vi "Create TCP Slave.vi"(8 "error in":errorcluster, 10 "port (502)":u16=502, 11 "address":string) -> (0 "error out":errorcluster, 3 "TCP slave instance":refnum<class "Modbus Slave.lvclass">)   [LabVIEW 2013, in "Modbus Library - Advance.lvlib" / "API Main.lvlib"]
doc: "Creates a standard TCP slave with an IP ADU. If the data model input is unwired, a standard data model will be initialized and used. If the input is wired, the code will check to make sure that it is not the default value for the class (it should be initialized). If the default value of the class is wired, the standard model will be initialized and used."
uses:
  API Main.lvlib
  Slave/Modbus Slave.lvclass
  Transmission Data Unit/IP/IP Data Unit.lvclass
  Network Protocol/Network Slave/TCP/TCP Slave.lvclass
  Transmission Data Unit/Transmission Data Unit.lvclass/Transmission Data Unit.ctl
  Super Data Model/Super Data Model.lvclass
  Network Protocol/Network Slave/TCP/TCP Slave.lvclass/TCP Slave.ctl
  Slave/Modbus Slave.lvclass/Modbus Slave.ctl
  Modbus API.lvclass/Modbus API.ctl
  Network Protocol/Network Slave/TCP/Write Port.vi
  Network Protocol/Network Slave/TCP/Write listening net address.vi
  <vilib>/Utility/error.llb/Clear Errors.vi
  Super Data Model/ShutDown.vi
  Modbus API.lvclass
  Transmission Data Unit/Transmission Data Unit.lvclass
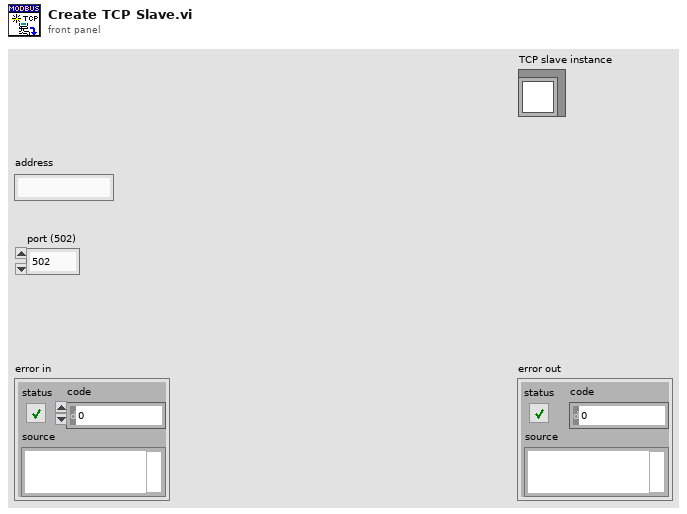
[diagram p1: front panel]
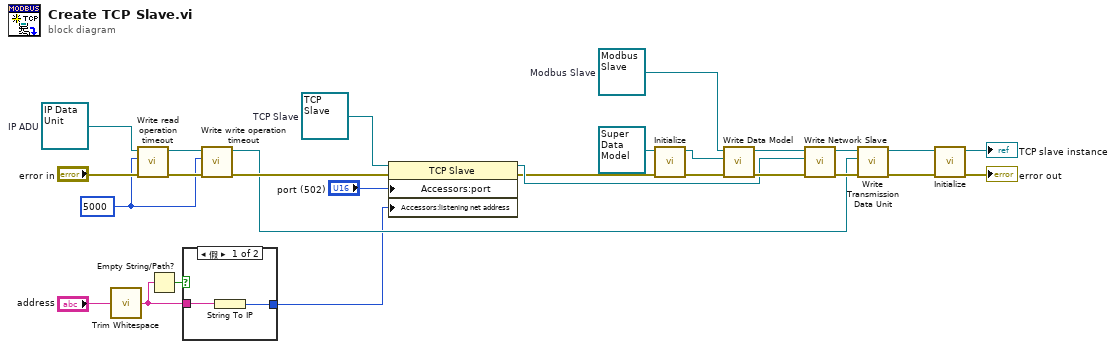
[diagram p0: block diagram]
diagram:
  w10 = 5000 ("read operation timeout")
  w27 = refnum<class "TCP Slave.lvclass"> refnum  # TCP Slave
  w12 = refnum<class "IP Data Unit.lvclass"> refnum  # IP ADU
  w23 = refnum<class "Modbus Slave.lvclass"> refnum  # Modbus Slave
  n1 = call <vilib>:"Trim Whitespace.vi"("string"="address") -> ("trimmed string"=w6:string)  [unwired: 1 in]
  n2 = call "Write read operation timeout.vi"("error in (no error)"="error in", "read operation timeout"=w10, "transmission data unit in"=w12) -> ("error out"=w14:errorcluster, "transmission data unit out"=w11:refnum<class "IP Data Unit.lvclass">)  [unwired: 7 in]
  n3 = Empty String/Path?(string/path=w6) -> (empty?=w7:bool)
  n4 = case shown="假" w7 {
    tunnel: w6 -> [w29 _]
    tunnel: [w28 _] -> w5
    frame False {
      n5 = String To IP(1:w29) -> (0:w28:u32)
    }
    frame True {
    }
  }
  n6 = call "Write write operation timeout.vi"("error in (no error)"=w14, "write operation timeout"=w10, "transmission data unit in"=w11) -> ("error out"=w15:errorcluster, "transmission data unit out"=w9:refnum<class "IP Data Unit.lvclass">)  [unwired: 7 in]
  n7 = property class="TCP Slave"(reference=w27, error in=w15, "Accessors:port"="port (502)", "Accessors:listening net address"=w5) -> (reference out=w16:refnum<class "TCP Slave.lvclass">, error out=w4:errorcluster)
  n8 = call "Initialize.vi"("错误输入（无错误）"=w4, "Super Data Model in"=refnum<class "Super Data Model.lvclass"> refnum) -> ("错误输出"=w2:errorcluster, "Super Data Model out"=w3:refnum<class "Super Data Model.lvclass">)  [unwired: 8 in]
  n9 = call "Write Data Model.vi"("error in"=w2, "Super Data Model"=w3, "Modbus slave in"=w23) -> ("error out"=w17:errorcluster, "Modbus slave out"=w19:refnum<class "Modbus Slave.lvclass">)  [unwired: 7 in]
  n10 = call "Write Network Slave.vi"("error in"=w17, "network slave"=w16, "Modbus slave in"=w19) -> ("error out"=w18:errorcluster, "Modbus slave out"=w20:refnum<class "Modbus Slave.lvclass">)  [unwired: 7 in]
  n11 = call "Write Transmission Data Unit.vi"("error in"=w18, "transmission data unit"=w9, "Modbus instance in"=w20) -> ("error out"=w21:errorcluster, "Modbus instance out"=w22:refnum<class "Modbus Slave.lvclass">)  [unwired: 7 in]
  n12 = call-dynamic "Initialize.vi"("error in"=w21, "Modbus slave in"=w22) -> ("error out"=→"error out":errorcluster, "Modbus slave out"=→"TCP slave instance":refnum<class "Modbus Slave.lvclass">)  [unwired: 8 in]
